vi "PolyFitDestVel.vi"(5 "TargetTime":dbl, 6 "use model?":bool, 7 "TargetPos":dbl[](array[numeric]), 8 "error in (no error)":errorcluster, 9 "robotModel":dbl[][](array[numeric])=array600x16[9600 elements], 10 "Robot":refnum<class "Robot.lvclass">, 11 "Utilities in":refnum<class "Utilities.lvclass">) -> (0 "error out":errorcluster, 2 "vf":dbl format="%.2f", 3 "Utilities out":refnum<class "Utilities.lvclass">)   [LabVIEW 2024, in "Utilities.lvclass"]
uses:
  Utilities.lvclass
  Robot_class/Robot.lvclass
  C:/Users/as119/OneDrive/Documentos/roboIME/SSL_AI/Object_class/Object.lvclass
  Robot_class/Robot.lvclass/Robot.ctl
  Object_class/Object.lvclass/Object.ctl
  <vilib>/Analysis/6fits.llb/Curve Fitting Criteria.ctl
  <vilib>/Analysis/6fits.llb/General Linear Fit Algorithm.ctl
  Robot_class/Read est_v_tang.vi
  Robot_class/Read est_v_norm.vi
  Object_class/Read position(x,y).vi
  <vilib>/Analysis/Matrix/Numeric/Conversions/Array To Matrix.vi
  <vilib>/Analysis/Matrix/Numeric/Conversions/Array To Matrix - RA2.vi
  <vilib>/Analysis/NI_AALPro.lvlib
  Game_class/Game.lvclass
panel:
  out "search_results":dbl[][](array[numeric])
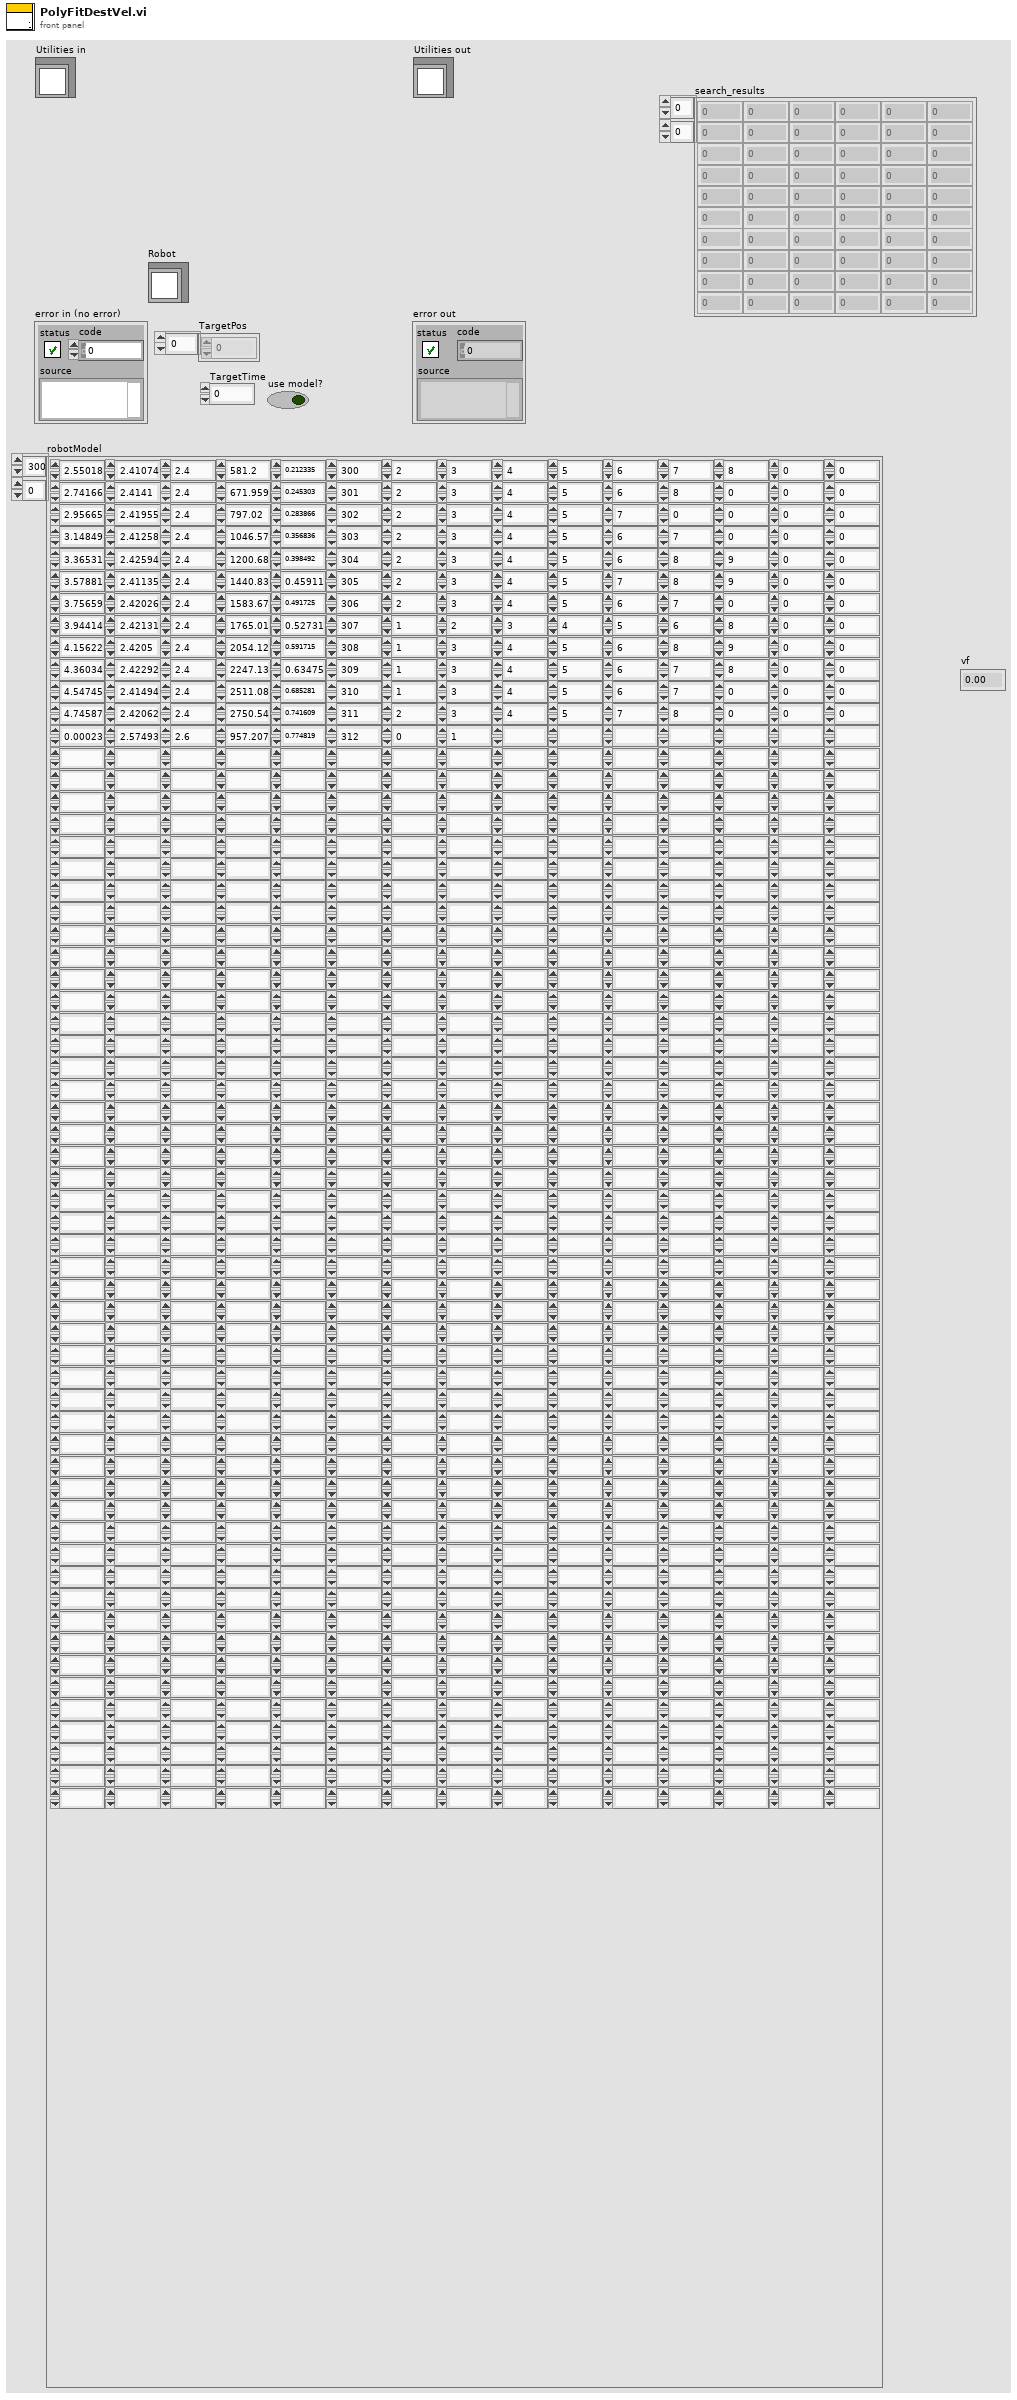
[diagram p1: front panel]
types:
  T1 = typedef "NI_AALPro.lvlib/General Linear Fit Algorithm.ctl" = u16
  T2 = typedef "NI_AALPro.lvlib/Curve Fitting Criteria.ctl" = u16
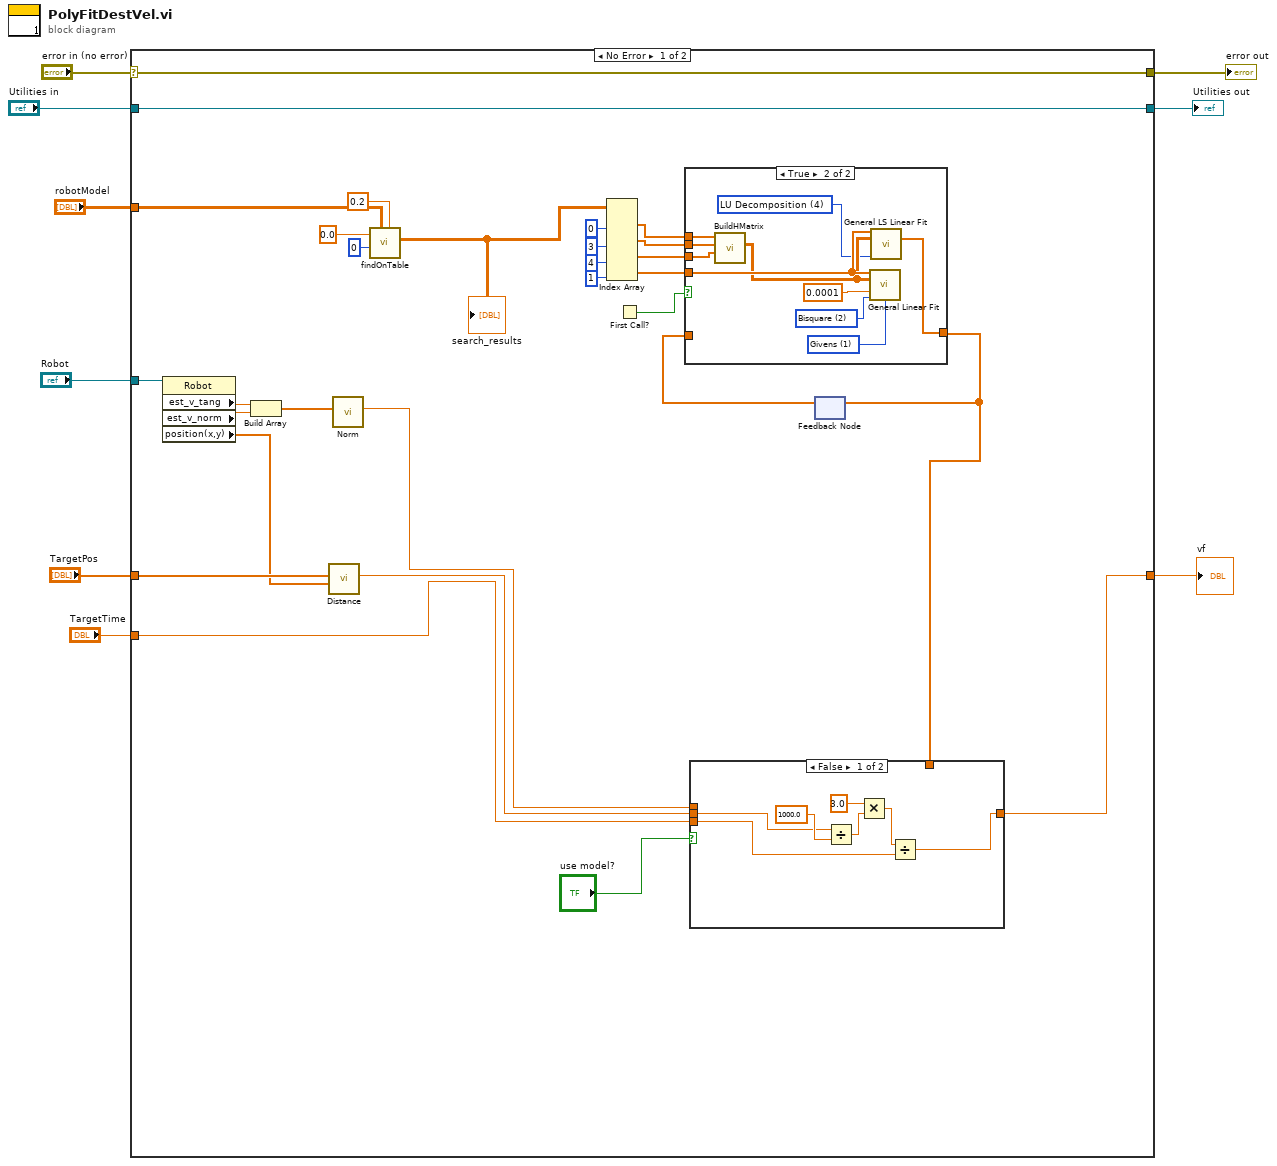
[diagram p0: block diagram]
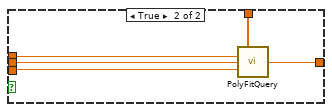
[diagram p2: hidden frame]
diagram:
  n1 = case shown="No Error" "error in (no error)" {
    selector: "error in (no error)" -> [w37 w63]
    tunnel: [w37 w63] -> w8
    tunnel: [w38 w62] -> w6
    tunnel: "Utilities in" -> [w38 w62]
    tunnel: "Robot" -> [w26 _]
    tunnel: "robotModel" -> [w20 _]
    tunnel: "TargetPos" -> [w23 _]
    tunnel: "TargetTime" -> [w10 _]
    tunnel: [w13 _] -> w1
    frame No Error {
      n2 = property class="Robot"(reference=w26) -> ("est_v_tang"=w25:dbl, "est_v_norm"=w24:dbl, "position(x,y)"=w21:dbl[])  [unwired: 1 in, 2 out]
      n3 = Build Array(w25, w24) -> (w22:dbl[])
      n4 = call "Distance.vi"("P1"=w21, "P2"=w23) -> ("Distance"=w11:dbl)  [unwired: 7 in, 2 out]
      n5 = call "Norm.vi"("2D vector"=w22) -> ("Modulo"=w12:dbl)  [unwired: 8 in, 2 out]
      n6 = call "findOnTable.vi"("delta"=0.2, "table"=w20, "column"=0, "key"=0.0) -> ("search_results"=w19:dbl[][])  [unwired: 5 in, 2 out]
      "search_results" <- w19
      n7 = Index Array(array=w19, index (col) #1=0 ("disabled index (col)"), index (col) #2=3 ("index (col)"), index (col) #3=4 ("index (col)"), index (col) #4=1 ("index (col)")) -> (element #1=w31:dbl[], element #2=w30:dbl[], element #3=w29:dbl[], element #4=w32:dbl[])  [unwired: 4 in]
      n8 = First Call?() -> (First Call?: T/F=w28:bool)
      n9 = feedback #1() -> (w27:dbl[])  [unwired: 1 in]
      n10 = case shown="True" w28 {
        tunnel: w32 -> [_ w56]
        tunnel: w31 -> [_ w61]
        tunnel: w30 -> [_ w60]
        tunnel: w29 -> [_ w59]
        tunnel: [w51 w52] -> w14
        tunnel: w27 -> [w51 _]
        frame False {
        }
        frame True {
          w53 = T1 4 items=["SVD", "Givens", "Givens2", "Householder", "LU Decomposition", "Cholesky", "SVD for Rank Deficient H"] ("algorithm")
          w58 = T1 1 items=["SVD", "Givens", "Givens2", "Householder", "LU Decomposition", "Cholesky", "SVD for Rank Deficient H"] ("algorithm")
          w54 = T2 2 items=["Least Square", "Least Absolute Residual", "Bisquare"] ("method")
          n11 = call "BuildHMatrix.vi"("Z"=w59, "Y"=w60, "X"=w61) -> ("H"=w55:dbl[][])  [unwired: 6 in, 2 out]
          n12 = call <vilib>:"General Linear Fit.vi"("Y"=w56, "H"=w55, "tolerance"=0.0001, "method"=w54, "algorithm"=w58) -> ()  [unwired: 5 in, 6 out]
          n13 = call <vilib>:"General LS Linear Fit.vi"("Y"=w56, "H"=w55, "algorithm"=w53) -> ("Coefficients"=w52:dbl[])  [unwired: 8 in, 4 out]
        }
      }
      n14 = case shown="False" "use model?" {
        tunnel: w14 -> [_ w50]
        tunnel: [w39 w49] -> w13
        tunnel: w12 -> [_ w48]
        tunnel: w11 -> [w41 w47]
        tunnel: w10 -> [w40 w46]
        frame False {
          n15 = Divide(x=w41, y=1000.0) -> (x/y=w42:dbl)
          n16 = Multiply(x=3.0, y=w42) -> (x*y=w44:dbl)
          n17 = Divide(x=w44, y=w40) -> (x/y=w39:dbl)
        }
        frame True {
          n18 = call "PolyFitQuery.vi"("Coefficients"=w50, "x"=w48, "y"=w47, "z"=w46) -> ("f(x, y, z)"=w49:dbl)  [unwired: 9 in, 2 out]
        }
      }
      n19 = feedback-in #1(w14) -> ()
    }
    frame Error {
    }
  }
  "error out" <- w8
  "Utilities out" <- w6
  "vf" <- w1
